vi "Test.vi"() -> ()   [LabVIEW 2016, in "Screen Switching.lvlib" / "Screen Switching.lvclass"]
uses:
  Screen Switching.lvclass
panel:
  in  "单选按钮":enum32{"单选选项1", "单选选项2"}(radio)
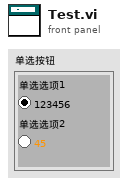
[diagram p1: front panel]
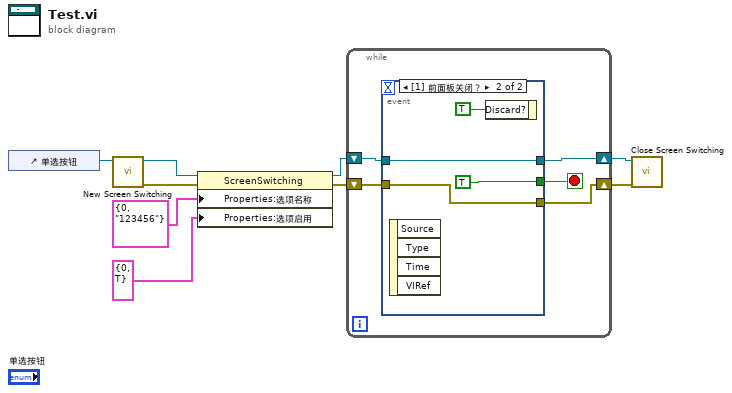
[diagram p0: block diagram]
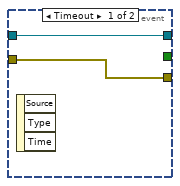
[diagram p2: hidden frame]
diagram:
  n1 = control-ref of="单选按钮"() -> (w9:refnum<vi>)
  n2 = call "New Screen Switching.vi"("Reference"=w9) -> ("error out"=w2:errorcluster, "ScreenSwitching out"=w8:refnum<class "Screen Switching.lvclass">)  [unwired: 9 in]
  n3 = property class="ScreenSwitching"(reference=w8, error in=w2, "Properties:选项名称"=cluster{"索引":i32, "名称":string} {"索引"=0, "名称"="123456"} ("选项名称"), "Properties:选项启用"=cluster{"索引":i32, "enable":bool} {"索引"=0, "enable"=TRUE} ("选项启用")) -> (reference out=w5:refnum<class "Screen Switching.lvclass">, error out=w3:errorcluster)
  n4 = while {
    shift-right: [w11] -> w6
    shift-left: w3 -> [w13]
    shift-right: [w12] -> w7
    shift-left: w5 -> [w14]
    stop <- w10 stop-if-true
    n5 = event shown="[1] 前面板关闭？" {
      selector: _ -> [_ _]
      dyn-events: _ -> [_ _]
      timeout: _ -> [_ _]
      tunnel: w14 -> [w16 w19]
      tunnel: w13 -> [w15 w18]
      tunnel: [w16 w19] -> w12
      tunnel: [w15 w18] -> w11
      tunnel: [_ TRUE] -> w10
      event Timeout {
        n6 = event-data() -> ()  [unwired: 1 in, 3 out]
      }
      event Panel Close? {
        n7 = event-data() -> ()  [unwired: 1 in, 4 out]
        n8 = event-data("Discard?"=TRUE ("放弃？")) -> ()  [unwired: 1 in, 1 out]
      }
    }
  }
  n9 = call "Close Screen Switching.vi"("error in (no error)"=w6, "ScreenSwitching in"=w7) -> ()  [unwired: 9 in, 1 out]
